vi "Connector Pane Pattern Reference.vi"() -> ()   [LabVIEW 2019]
doc: "This VI shows the connector pane index for each terminal for a given connector pane pattern.\nConnector panes can be rotated, which is why there are three patterns per connector pane number."
panel:
  out "Connector Pane Pattern Information":T1(array[cluster])=[{"Pattern"=4800, "Terminal Rects"=[{"Left"=0, "Top"=0, "Right"=32, "Bottom"=32}], "Pattern Images"=bytes[360]}, {"Pattern"=4801, "Terminal Rects"=[{"Left"=16, "Top"=0, "Right"=32, "Bottom"=32}, {"Left"=0, "Top"=0, "Right"=16, "Bottom"=32}], "Pattern Images"=bytes[720]}, {"Pattern"=4802, "Terminal Rects"=[{"Left"=16, "Top"=0, "Right"=32, "Bottom"=32}, {"Left"=0, "Top"=16, "Right"=16, "Bottom"=32}, {"Left"=0, "Top"=0, "Right"=16, "Bottom"=16}], "Pattern Images"=bytes[1080]}, {"Pattern"=4803, "Terminal Rects"=[{"Left"=0, "Top"=21, "Right"=32, "Bottom"=32}, {"Left"=0, "Top"=11, "Right"=32, "Bottom"=21}, {"Left"=0, "Top"=0, "Right"=32, "Bottom"=11}], "Pattern Images"=bytes[1080]}, {"Pattern"=4804, "Terminal Rects"=[{"Left"=16, "Top"=0, "Right"=32, "Bottom"=32}, {"Left"=0, "Top"=21, "Right"=16, "Bottom"=32}, {"Left"=0, "Top"=11, "Right"=16, "Bottom"=21}, {"Left"=0, "Top"=0, "Right"=16, "Bottom"=11}], "Pattern Images"=bytes[1440]}, {"Pattern"=4805, "Terminal Rects"=[{"Left"=16, "Top"=16, "Right"=32, "Bottom"=32}, {"Left"=16, "Top"=0, "Right"=32, "Bottom"=16}, {"Left"=0, "Top"=16, "Right"=16, "Bottom"=32}, {"Left"=0, "Top"=0, "Right"=16, "Bottom"=16}], "Pattern Images"=bytes[1440]}, {"Pattern"=4806, "Terminal Rects"=[{"Left"=0, "Top"=24, "Right"=32, "Bottom"=32}, {"Left"=0, "Top"=16, "Right"=32, "Bottom"=24}, {"Left"=0, "Top"=8, "Right"=32, "Bottom"=16}, {"Left"=0, "Top"=0, "Right"=32, "Bottom"=8}], "Pattern Images"=bytes[1440]}, {"Pattern"=4807, "Terminal Rects"=[{"Left"=16, "Top"=16, "Right"=32, "Bottom"=32}, {"Left"=16, "Top"=0, "Right"=32, "Bottom"=16}, {"Left"=0, "Top"=21, "Right"=16, "Bottom"=32}, {"Left"=0, "Top"=11, "Right"=16, "Bottom"=21}, {"Left"=0, "Top"=0, "Right"=16, "Bottom"=11}], "Pattern Images"=bytes[1800]}, {"Pattern"=4808, "Terminal Rects"=[{"Left"=16, "Top"=0, "Right"=32, "Bottom"=32}, {"Left"=0, "Top"=24, "Right"=16, "Bottom"=32}, {"Left"=0, "Top"=16, "Right"=16, "Bottom"=24}, {"Left"=0, "Top"=8, "Right"=16, "Bottom"=16}, {"Left"=0, "Top"=0, "Right"=16, "Bottom"=8}], "Pattern Images"=bytes[1800]}, {"Pattern"=4809, "Terminal Rects"=[{"Left"=16, "Top"=16, "Right"=32, "Bottom"=32}, {"Left"=16, "Top"=0, "Right"=32, "Bottom"=16}, {"Left"=0, "Top"=24, "Right"=16, "Bottom"=32}, {"Left"=0, "Top"=16, "Right"=16, "Bottom"=24}, {"Left"=0, "Top"=8, "Right"=16, "Bottom"=16}, {"Left"=0, "Top"=0, "Right"=16, "Bottom"=8}], "Pattern Images"=bytes[2160]}, {"Pattern"=4810, "Terminal Rects"=[{"Left"=16, "Top"=21, "Right"=32, "Bottom"=32}, {"Left"=16, "Top"=11, "Right"=32, "Bottom"=21}, {"Left"=16, "Top"=0, "Right"=32, "Bottom"=11}, {"Left"=0, "Top"=21, "Right"=16, "Bottom"=32}, {"Left"=0, "Top"=11, "Right"=16, "Bottom"=21}, {"Left"=0, "Top"=0, "Right"=16, "Bottom"=11}], "Pattern Images"=bytes[2160]}, {"Pattern"=4811, "Terminal Rects"=[{"Left"=16, "Top"=21, "Right"=32, "Bottom"=32}, {"Left"=16, "Top"=11, "Right"=32, "Bottom"=21}, {"Left"=16, "Top"=0, "Right"=32, "Bottom"=11}, {"Left"=0, "Top"=24, "Right"=16, "Bottom"=32}, {"Left"=0, "Top"=16, "Right"=16, "Bottom"=24}, {"Left"=0, "Top"=8, "Right"=16, "Bottom"=16}, {"Left"=0, "Top"=0, "Right"=16, "Bottom"=8}], "Pattern Images"=bytes[2520]}, {"Pattern"=4812, "Terminal Rects"=[{"Left"=16, "Top"=24, "Right"=32, "Bottom"=32}, {"Left"=16, "Top"=16, "Right"=32, "Bottom"=24}, {"Left"=16, "Top"=8, "Right"=32, "Bottom"=16}, {"Left"=16, "Top"=0, "Right"=32, "Bottom"=8}, {"Left"=0, "Top"=24, "Right"=16, "Bottom"=32}, {"Left"=0, "Top"=16, "Right"=16, "Bottom"=24}, {"Left"=0, "Top"=8, "Right"=16, "Bottom"=16}, {"Left"=0, "Top"=0, "Right"=16, "Bottom"=8}], "Pattern Images"=bytes[2880]}, {"Pattern"=4813, "Terminal Rects"=[{"Left"=16, "Top"=24, "Right"=32, "Bottom"=32}, {"Left"=16, "Top"=16, "Right"=32, "Bottom"=24}, {"Left"=16, "Top"=8, "Right"=32, "Bottom"=16}, {"Left"=16, "Top"=0, "Right"=32, "Bottom"=8}, {"Left"=8, "Top"=0, "Right"=16, "Bottom"=32}, {"Left"=0, "Top"=24, "Right"=8, "Bottom"=32}, {"Left"=0, "Top"=16, "Right"=8, "Bottom"=24}, {"Left"=0, "Top"=8, "Right"=8, "Bottom"=16}, {"Left"=0, "Top"=0, "Right"=8, "Bottom"=8}], "Pattern Images"=bytes[3240]}, {"Pattern"=4814, "Terminal Rects"=[{"Left"=16, "Top"=24, "Right"=32, "Bottom"=32}, {"Left"=16, "Top"=16, "Right"=32, "Bottom"=24}, {"Left"=16, "Top"=8, "Right"=32, "Bottom"=16}, {"Left"=16, "Top"=0, "Right"=32, "Bottom"=8}, {"Left"=8, "Top"=16, "Right"=16, "Bottom"=32}, {"Left"=8, "Top"=0, "Right"=16, "Bottom"=16}, {"Left"=0, "Top"=24, "Right"=8, "Bottom"=32}, {"Left"=0, "Top"=16, "Right"=8, "Bottom"=24}, {"Left"=0, "Top"=8, "Right"=8, "Bottom"=16}, {"Left"=0, "Top"=0, "Right"=8, "Bottom"=8}], "Pattern Images"=bytes[3600]}, {"Pattern"=4815, "Terminal Rects"=[{"Left"=24, "Top"=24, "Right"=32, "Bottom"=32}, {"Left"=24, "Top"=16, "Right"=32, "Bottom"=24}, {"Left"=24, "Top"=8, "Right"=32, "Bottom"=16}, {"Left"=24, "Top"=0, "Right"=32, "Bottom"=8}, {"Left"=16, "Top"=16, "Right"=24, "Bottom"=32}, {"Left"=16, "Top"=0, "Right"=24, "Bottom"=16}, {"Left"=8, "Top"=16, "Right"=16, "Bottom"=32}, {"Left"=8, "Top"=0, "Right"=16, "Bottom"=16}, {"Left"=0, "Top"=24, "Right"=8, "Bottom"=32}, {"Left"=0, "Top"=16, "Right"=8, "Bottom"=24}, {"Left"=0, "Top"=8, "Right"=8, "Bottom"=16}, {"Left"=0, "Top"=0, "Right"=8, "Bottom"=8}], "Pattern Images"=bytes[4320]}, {"Pattern"=4816, "Terminal Rects"=[{"Left"=0, "Top"=0, "Right"=8, "Bottom"=11}, {"Left"=8, "Top"=0, "Right"=16, "Bottom"=11}, {"Left"=0, "Top"=11, "Right"=16, "Bottom"=21}, {"Left"=0, "Top"=21, "Right"=8, "Bottom"=32}, {"Left"=8, "Top"=21, "Right"=16, "Bottom"=32}, {"Left"=16, "Top"=0, "Right"=32, "Bottom"=32}], "Pattern Images"=bytes[2160]}, {"Pattern"=4817, "Terminal Rects"=[{"Left"=0, "Top"=0, "Right"=8, "Bottom"=11}, {"Left"=8, "Top"=0, "Right"=16, "Bottom"=11}, {"Left"=0, "Top"=11, "Right"=16, "Bottom"=21}, {"Left"=0, "Top"=21, "Right"=8, "Bottom"=32}, {"Left"=8, "Top"=21, "Right"=16, "Bottom"=32}, {"Left"=16, "Top"=0, "Right"=32, "Bottom"=16}, {"Left"=16, "Top"=16, "Right"=32, "Bottom"=32}], "Pattern Images"=bytes[2520]}, {"Pattern"=4818, "Terminal Rects"=[{"Left"=0, "Top"=0, "Right"=8, "Bottom"=11}, {"Left"=8, "Top"=0, "Right"=16, "Bottom"=11}, {"Left"=0, "Top"=11, "Right"=16, "Bottom"=21}, {"Left"=0, "Top"=21, "Right"=8, "Bottom"=32}, {"Left"=8, "Top"=21, "Right"=16, "Bottom"=32}, {"Left"=16, "Top"=0, "Right"=32, "Bottom"=11}, {"Left"=16, "Top"=11, "Right"=32, "Bottom"=21}, {"Left"=16, "Top"=21, "Right"=32, "Bottom"=32}], "Pattern Images"=bytes[2880]}, {"Pattern"=4819, "Terminal Rects"=[{"Left"=0, "Top"=0, "Right"=8, "Bottom"=11}, {"Left"=8, "Top"=0, "Right"=16, "Bottom"=11}, {"Left"=0, "Top"=11, "Right"=16, "Bottom"=21}, {"Left"=0, "Top"=21, "Right"=8, "Bottom"=32}, {"Left"=8, "Top"=21, "Right"=16, "Bottom"=32}, {"Left"=16, "Top"=0, "Right"=32, "Bottom"=8}, {"Left"=16, "Top"=8, "Right"=32, "Bottom"=16}, {"Left"=16, "Top"=16, "Right"=32, "Bottom"=24}, {"Left"=16, "Top"=24, "Right"=32, "Bottom"=32}], "Pattern Images"=bytes[3240]}, {"Pattern"=4820, "Terminal Rects"=[{"Left"=0, "Top"=0, "Right"=8, "Bottom"=11}, {"Left"=8, "Top"=0, "Right"=16, "Bottom"=11}, {"Left"=0, "Top"=11, "Right"=16, "Bottom"=21}, {"Left"=0, "Top"=21, "Right"=8, "Bottom"=32}, {"Left"=8, "Top"=21, "Right"=16, "Bottom"=32}, {"Left"=16, "Top"=0, "Right"=24, "Bottom"=11}, {"Left"=24, "Top"=0, "Right"=32, "Bottom"=11}, {"Left"=16, "Top"=11, "Right"=32, "Bottom"=21}, {"Left"=16, "Top"=21, "Right"=24, "Bottom"=32}, {"Left"=24, "Top"=21, "Right"=32, "Bottom"=32}], "Pattern Images"=bytes[3600]}, {"Pattern"=4821, "Terminal Rects"=[{"Left"=0, "Top"=0, "Right"=8, "Bottom"=11}, {"Left"=8, "Top"=0, "Right"=16, "Bottom"=11}, {"Left"=0, "Top"=11, "Right"=16, "Bottom"=21}, {"Left"=0, "Top"=21, "Right"=8, "Bottom"=32}, {"Left"=8, "Top"=21, "Right"=16, "Bottom"=32}, {"Left"=16, "Top"=0, "Right"=24, "Bottom"=16}, {"Left"=24, "Top"=0, "Right"=32, "Bottom"=8}, {"Left"=24, "Top"=8, "Right"=32, "Bottom"=16}, {"Left"=16, "Top"=16, "Right"=24, "Bottom"=32}, {"Left"=24, "Top"=16, "Right"=32, "Bottom"=24}, {"Left"=24, "Top"=24, "Right"=32, "Bottom"=32}], "Pattern Images"=bytes[3960]}, {"Pattern"=4822, "Terminal Rects"=[{"Left"=0, "Top"=0, "Right"=8, "Bottom"=8}, {"Left"=8, "Top"=0, "Right"=16, "Bottom"=16}, {"Left"=0, "Top"=8, "Right"=8, "Bottom"=16}, {"Left"=0, "Top"=16, "Right"=8, "Bottom"=24}, {"Left"=8, "Top"=16, "Right"=16, "Bottom"=32}, {"Left"=0, "Top"=24, "Right"=8, "Bottom"=32}, {"Left"=16, "Top"=0, "Right"=32, "Bottom"=11}, {"Left"=16, "Top"=11, "Right"=32, "Bottom"=21}, {"Left"=16, "Top"=21, "Right"=32, "Bottom"=32}], "Pattern Images"=bytes[3240]}, {"Pattern"=4823, "Terminal Rects"=[{"Left"=0, "Top"=0, "Right"=8, "Bottom"=8}, {"Left"=0, "Top"=8, "Right"=8, "Bottom"=16}, {"Left"=0, "Top"=16, "Right"=8, "Bottom"=24}, {"Left"=0, "Top"=24, "Right"=8, "Bottom"=32}, {"Left"=8, "Top"=0, "Right"=16, "Bottom"=32}, {"Left"=16, "Top"=0, "Right"=32, "Bottom"=32}], "Pattern Images"=bytes[2160]}, {"Pattern"=4824, "Terminal Rects"=[{"Left"=0, "Top"=0, "Right"=8, "Bottom"=8}, {"Left"=0, "Top"=8, "Right"=8, "Bottom"=16}, {"Left"=0, "Top"=16, "Right"=8, "Bottom"=24}, {"Left"=0, "Top"=24, "Right"=8, "Bottom"=32}, {"Left"=8, "Top"=0, "Right"=16, "Bottom"=32}, {"Left"=16, "Top"=0, "Right"=32, "Bottom"=16}, {"Left"=16, "Top"=16, "Right"=32, "Bottom"=32}], "Pattern Images"=bytes[2520]}, {"Pattern"=4825, "Terminal Rects"=[{"Left"=0, "Top"=0, "Right"=8, "Bottom"=8}, {"Left"=0, "Top"=8, "Right"=8, "Bottom"=16}, {"Left"=0, "Top"=16, "Right"=8, "Bottom"=24}, {"Left"=0, "Top"=24, "Right"=8, "Bottom"=32}, {"Left"=8, "Top"=0, "Right"=16, "Bottom"=32}, {"Left"=16, "Top"=0, "Right"=32, "Bottom"=11}, {"Left"=16, "Top"=11, "Right"=32, "Bottom"=21}, {"Left"=16, "Top"=21, "Right"=32, "Bottom"=32}], "Pattern Images"=bytes[2880]}, {"Pattern"=4826, "Terminal Rects"=[{"Left"=24, "Top"=24, "Right"=32, "Bottom"=32}, {"Left"=24, "Top"=16, "Right"=32, "Bottom"=24}, {"Left"=24, "Top"=8, "Right"=32, "Bottom"=16}, {"Left"=24, "Top"=0, "Right"=32, "Bottom"=8}, {"Left"=16, "Top"=0, "Right"=24, "Bottom"=32}, {"Left"=8, "Top"=0, "Right"=16, "Bottom"=32}, {"Left"=0, "Top"=24, "Right"=8, "Bottom"=32}, {"Left"=0, "Top"=16, "Right"=8, "Bottom"=24}, {"Left"=0, "Top"=8, "Right"=8, "Bottom"=16}, {"Left"=0, "Top"=0, "Right"=8, "Bottom"=8}], "Pattern Images"=bytes[3600]}, {"Pattern"=4827, "Terminal Rects"=[{"Left"=16, "Top"=0, "Right"=32, "Bottom"=32}, {"Left"=8, "Top"=16, "Right"=16, "Bottom"=32}, {"Left"=8, "Top"=0, "Right"=16, "Bottom"=16}, {"Left"=0, "Top"=24, "Right"=8, "Bottom"=32}, {"Left"=0, "Top"=16, "Right"=8, "Bottom"=24}, {"Left"=0, "Top"=8, "Right"=8, "Bottom"=16}, {"Left"=0, "Top"=0, "Right"=8, "Bottom"=8}], "Pattern Images"=bytes[2520]}, {"Pattern"=4828, "Terminal Rects"=[{"Left"=16, "Top"=16, "Right"=32, "Bottom"=32}, {"Left"=16, "Top"=0, "Right"=32, "Bottom"=16}, {"Left"=8, "Top"=16, "Right"=16, "Bottom"=32}, {"Left"=8, "Top"=0, "Right"=16, "Bottom"=16}, {"Left"=0, "Top"=24, "Right"=8, "Bottom"=32}, {"Left"=0, "Top"=16, "Right"=8, "Bottom"=24}, {"Left"=0, "Top"=8, "Right"=8, "Bottom"=16}, {"Left"=0, "Top"=0, "Right"=8, "Bottom"=8}], "Pattern Images"=bytes[2880]}, {"Pattern"=4829, "Terminal Rects"=[{"Left"=24, "Top"=24, "Right"=32, "Bottom"=32}, {"Left"=24, "Top"=16, "Right"=32, "Bottom"=24}, {"Left"=24, "Top"=8, "Right"=32, "Bottom"=16}, {"Left"=24, "Top"=0, "Right"=32, "Bottom"=8}, {"Left"=16, "Top"=0, "Right"=24, "Bottom"=32}, {"Left"=8, "Top"=16, "Right"=16, "Bottom"=32}, {"Left"=8, "Top"=0, "Right"=16, "Bottom"=16}, {"Left"=0, "Top"=24, "Right"=8, "Bottom"=32}, {"Left"=0, "Top"=16, "Right"=8, "Bottom"=24}, {"Left"=0, "Top"=8, "Right"=8, "Bottom"=16}, {"Left"=0, "Top"=0, "Right"=8, "Bottom"=8}], "Pattern Images"=bytes[3960]}, {"Pattern"=4830, "Terminal Rects"=[{"Left"=21, "Top"=0, "Right"=32, "Bottom"=32}, {"Left"=11, "Top"=0, "Right"=21, "Bottom"=32}, {"Left"=0, "Top"=16, "Right"=11, "Bottom"=32}, {"Left"=0, "Top"=0, "Right"=11, "Bottom"=16}], "Pattern Images"=bytes[1440]}, {"Pattern"=4831, "Terminal Rects"=[{"Left"=21, "Top"=0, "Right"=32, "Bottom"=32}, {"Left"=11, "Top"=0, "Right"=21, "Bottom"=32}, {"Left"=0, "Top"=21, "Right"=11, "Bottom"=32}, {"Left"=0, "Top"=11, "Right"=11, "Bottom"=21}, {"Left"=0, "Top"=0, "Right"=11, "Bottom"=11}], "Pattern Images"=bytes[1800]}, {"Pattern"=4832, "Terminal Rects"=[{"Left"=21, "Top"=16, "Right"=32, "Bottom"=32}, {"Left"=21, "Top"=0, "Right"=32, "Bottom"=16}, {"Left"=11, "Top"=0, "Right"=21, "Bottom"=32}, {"Left"=0, "Top"=21, "Right"=11, "Bottom"=32}, {"Left"=0, "Top"=11, "Right"=11, "Bottom"=21}, {"Left"=0, "Top"=0, "Right"=11, "Bottom"=11}], "Pattern Images"=bytes[2160]}, {"Pattern"=4833, "Terminal Rects"=[{"Left"=0, "Top"=0, "Right"=7, "Bottom"=7}, {"Left"=7, "Top"=0, "Right"=13, "Bottom"=16}, {"Left"=13, "Top"=0, "Right"=19, "Bottom"=16}, {"Left"=19, "Top"=0, "Right"=25, "Bottom"=16}, {"Left"=25, "Top"=0, "Right"=32, "Bottom"=7}, {"Left"=0, "Top"=7, "Right"=7, "Bottom"=13}, {"Left"=25, "Top"=7, "Right"=32, "Bottom"=13}, {"Left"=0, "Top"=13, "Right"=7, "Bottom"=19}, {"Left"=25, "Top"=13, "Right"=32, "Bottom"=19}, {"Left"=0, "Top"=19, "Right"=7, "Bottom"=25}, {"Left"=25, "Top"=19, "Right"=32, "Bottom"=25}, {"Left"=0, "Top"=25, "Right"=7, "Bottom"=32}, {"Left"=7, "Top"=16, "Right"=13, "Bottom"=32}, {"Left"=13, "Top"=16, "Right"=19, "Bottom"=32}, {"Left"=19, "Top"=16, "Right"=25, "Bottom"=32}, {"Left"=25, "Top"=25, "Right"=32, "Bottom"=32}], "Pattern Images"=bytes[5760]}, {"Pattern"=4834, "Terminal Rects"=[{"Left"=0, "Top"=0, "Right"=6, "Bottom"=6}, {"Left"=0, "Top"=6, "Right"=6, "Bottom"=11}, {"Left"=0, "Top"=11, "Right"=6, "Bottom"=16}, {"Left"=0, "Top"=16, "Right"=6, "Bottom"=21}, {"Left"=0, "Top"=21, "Right"=6, "Bottom"=26}, {"Left"=0, "Top"=26, "Right"=6, "Bottom"=32}, {"Left"=6, "Top"=0, "Right"=11, "Bottom"=16}, {"Left"=6, "Top"=16, "Right"=11, "Bottom"=32}, {"Left"=11, "Top"=0, "Right"=16, "Bottom"=16}, {"Left"=11, "Top"=16, "Right"=16, "Bottom"=32}, {"Left"=16, "Top"=0, "Right"=21, "Bottom"=16}, {"Left"=16, "Top"=16, "Right"=21, "Bottom"=32}, {"Left"=21, "Top"=0, "Right"=26, "Bottom"=16}, {"Left"=21, "Top"=16, "Right"=26, "Bottom"=32}, {"Left"=26, "Top"=0, "Right"=32, "Bottom"=6}, {"Left"=26, "Top"=6, "Right"=32, "Bottom"=11}, {"Left"=26, "Top"=11, "Right"=32, "Bottom"=16}, {"Left"=26, "Top"=16, "Right"=32, "Bottom"=21}, {"Left"=26, "Top"=21, "Right"=32, "Bottom"=26}, {"Left"=26, "Top"=26, "Right"=32, "Bottom"=32}], "Pattern Images"=bytes[7200]}, {"Pattern"=4835, "Terminal Rects"=[{"Left"=0, "Top"=0, "Right"=4, "Bottom"=4}, {"Left"=0, "Top"=4, "Right"=4, "Bottom"=8}, {"Left"=0, "Top"=8, "Right"=4, "Bottom"=12}, {"Left"=0, "Top"=12, "Right"=4, "Bottom"=16}, {"Left"=0, "Top"=16, "Right"=4, "Bottom"=20}, {"Left"=0, "Top"=20, "Right"=4, "Bottom"=24}, {"Left"=0, "Top"=24, "Right"=4, "Bottom"=28}, {"Left"=0, "Top"=28, "Right"=4, "Bottom"=32}, {"Left"=4, "Top"=0, "Right"=8, "Bottom"=16}, {"Left"=4, "Top"=16, "Right"=8, "Bottom"=32}, {"Left"=8, "Top"=0, "Right"=12, "Bottom"=16}, {"Left"=8, "Top"=16, "Right"=12, "Bottom"=32}, {"Left"=12, "Top"=0, "Right"=16, "Bottom"=16}, {"Left"=12, "Top"=16, "Right"=16, "Bottom"=32}, {"Left"=16, "Top"=0, "Right"=20, "Bottom"=16}, {"Left"=16, "Top"=16, "Right"=20, "Bottom"=32}, {"Left"=20, "Top"=0, "Right"=24, "Bottom"=16}, {"Left"=20, "Top"=16, "Right"=24, "Bottom"=32}, {"Left"=24, "Top"=0, "Right"=28, "Bottom"=16}, {"Left"=24, "Top"=16, "Right"=28, "Bottom"=32}, {"Left"=28, "Top"=0, "Right"=32, "Bottom"=4}, {"Left"=28, "Top"=4, "Right"=32, "Bottom"=8}, {"Left"=28, "Top"=8, "Right"=32, "Bottom"=12}, {"Left"=28, "Top"=12, "Right"=32, "Bottom"=16}, {"Left"=28, "Top"=16, "Right"=32, "Bottom"=20}, {"Left"=28, "Top"=20, "Right"=32, "Bottom"=24}, {"Left"=28, "Top"=24, "Right"=32, "Bottom"=28}, {"Left"=28, "Top"=28, "Right"=32, "Bottom"=32}], "Pattern Images"=bytes[10080]}]
  # "Overview: Provides information for manipulating VI Connector Panes through VI Scripting.\nInstructions:\nScroll through the array below to see terminal information for all possible VI connector pane patterns. The Pattern value in the array below corresponds to the \"Pattern\" property of the ConnectorPane class in VI Scripting. Note that connector panes can be rotated, which is why there are three images per pattern."
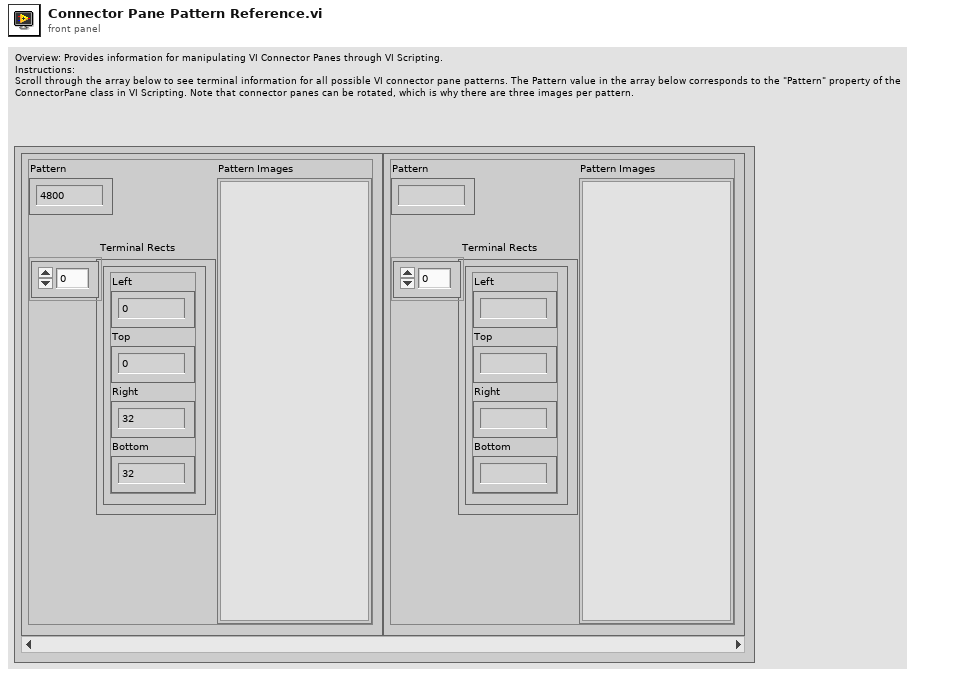
[diagram p1: front panel]
types:
  T1 = cluster{"Pattern":u32, "Terminal Rects":cluster{"Left":i64, "Top":i64, "Right":i64, "Bottom":i64}[], "Pattern Images":picture}[]
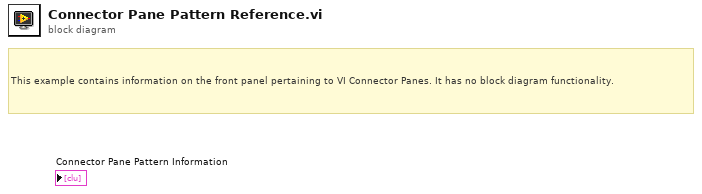
[diagram p0: block diagram]
diagram:
  # "This example contains information on the front panel pertaining to VI Connector Panes. It has no block diagram functionality."
